vi "new_get_opinion.vi"(10 "Axis":enum16{"X", "Y", "Z"}(ring), 11 "Mode":enum16{"Forward Pass", "Testing"}(ring)) -> (3 "opinons":dbl[](array[numeric]))   [LabVIEW 2014]
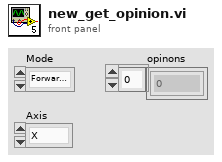
[diagram p1: front panel]
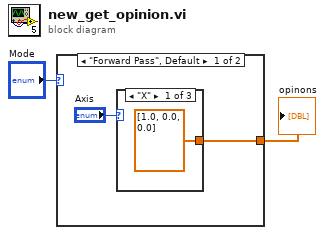
[diagram p0: block diagram]
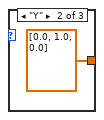
[diagram p2: hidden frame]
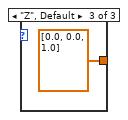
[diagram p3: hidden frame]
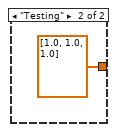
[diagram p4: hidden frame]
diagram:
  n1 = case shown="\"Forward Pass\", Default" "Mode" {
    tunnel: [w3 dbl[] [1.0, 1.0, 1.0] ("opinons")] -> w2
    frame "Forward Pass", Default {
      n2 = case shown="\"X\"" "Axis" {
        tunnel: [dbl[] [1.0, 0.0, 0.0] ("opinons") dbl[] [0.0, 1.0, 0.0] ("opinons") dbl[] [0.0, 0.0, 1.0] ("opinons")] -> w3
        frame "X" {
        }
        frame "Y" {
        }
        frame "Z", Default {
        }
      }
    }
    frame "Testing" {
    }
  }
  "opinons" <- w2
